vi "Global_variables.vi"() -> ()   [LabVIEW 2018]
panel:
  out "N Errors":dbl
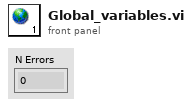
[diagram p1: front panel]
diagram:
